vi "Update Ack Flags.vi"(8 "error in (no error)":errorcluster, 10 "Cmd Value":bool[](array[boolean])=[FALSE, FALSE, FALSE, FALSE, FALSE, FALSE, FALSE, FALSE, FALSE, FALSE, FALSE, FALSE, FALSE, FALSE, FALSE, FALSE, TRUE, TRUE, TRUE, TRUE, TRUE, TRUE, TRUE, TRUE, TRUE, TRUE, TRUE, TRUE, TRUE, TRUE, TRUE, TRUE, TRUE, TRUE, TRUE], 11 "Value":bool) -> (0 "Error Out":errorcluster)   [LabVIEW 2018]
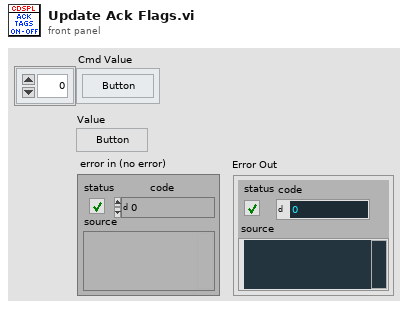
[diagram p1: front panel]
types:
  T1 = enum16{"Lamp A1", "Lamp B1", "Lamp C1", "Lamp D1", "Lamp E1", "Lamp F1", "Lamp G1", "Lamp H1", "Lamp A2", "Lamp B2", "Lamp C2", "Lamp D2", "Lamp E2", "Lamp F2", "Lamp G2", "Lamp H2", "Ack A1", "Ack B1", "Ack C1", "Ack D1", "Ack E1", "Ack F1", "Ack G1", "Ack H1", "Ack A2", "Ack B2", "Ack C2", "Ack D2", "Ack E2", "Ack F2", "Ack G2", "Ack H2", "SSM", "SAS", "LSM", ""}
  T2 = enum16{"Lamp A1", "Lamp B1", "Lamp C1", "Lamp D1", "Lamp E1", "Lamp F1", "Lamp G1", "Lamp H1", "Lamp A2", "Lamp B2", "Lamp C2", "Lamp D2", "Lamp E2", "Lamp F2", "Lamp G2", "Lamp H2", "Ack A1", "Ack B1", "Ack C1", "Ack D1", "Ack E1", "Ack F1", "Ack G1", "Ack H1", "Ack A2", "Ack B2", "Ack C2", "Ack D2", "Ack E2", "Ack F2", "Ack G2", "Ack H2", "SSM", "SAS", "LSM", ""}[]
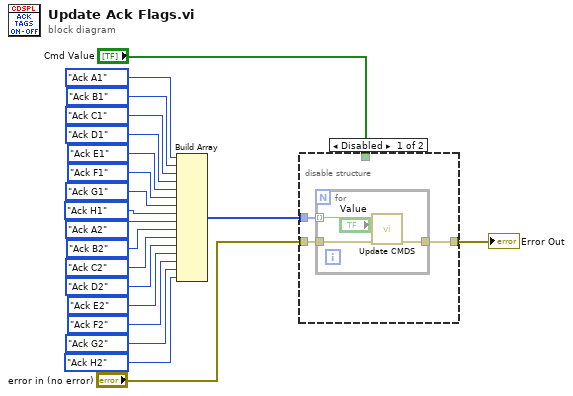
[diagram p0: block diagram]
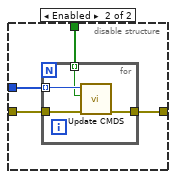
[diagram p2: hidden frame]
diagram:
  n1 = Build Array(T1."Ack A1" ("Tag"), T1."Ack B1" ("Tag"), T1."Ack C1" ("Tag"), T1."Ack D1" ("Tag"), T1."Ack E1" ("Tag"), T1."Ack F1" ("Tag"), T1."Ack G1" ("Tag"), T1."Ack H1" ("Tag"), T1."Ack A2" ("Tag"), T1."Ack B2" ("Tag"), T1."Ack C2" ("Tag"), T1."Ack D2" ("Tag"), T1."Ack E2" ("Tag"), T1."Ack F2" ("Tag"), T1."Ack G2" ("Tag"), T1."Ack H2" ("Tag")) -> (w4:T2)
  n2 = disable-structure shown="Disabled" {
    disable-tunnel: w4 -> [w23 w31]
    disable-tunnel: "error in (no error)" -> [w22 w30]
    disable-tunnel: [w21 w29] -> w2
    disable-tunnel: "Cmd Value" -> [_ w28]
    frame Disabled {
      n3 = for {
        tunnel: w23 -> [w27] mode=indexing
        tunnel: w22 -> [w25]
        tunnel: [w24] -> w21
        n4 = call "Update CMDS.vi"("error in (no error)"=w25, "New Value"="Value", "Tag"=w27) -> ("error out"=w24:errorcluster)  [unwired: 8 in]
      }
    }
    frame Enabled {
      n5 = for {
        tunnel: w31 -> [w35] mode=indexing
        tunnel: w30 -> [w34]
        tunnel: [w33] -> w29
        tunnel: w28 -> [w32] mode=indexing
        n6 = call "Update CMDS.vi"("error in (no error)"=w34, "New Value"=w32, "Tag"=w35) -> ("error out"=w33:errorcluster)  [unwired: 8 in]
      }
    }
  }
  "Error Out" <- w2
